vi "Get Switch Heater.vi"(2 "error in":T2, 3 "Communications Config":T1={"GPIB address"=22, "GPIB bus"=0, "connection ID"=refnum, "IP"="192.168.2.200", "Active Comm Interface"=0, "Serial Port"="", "Programmer Type"=0} {"Programmer Type" items=["Model 430", "Model 420"]; "Active Comm Interface" items=["TCP/IP (Model 430 Only)", "RS232", "IEEE488"]}) -> (0 "error out":T2, 1 "Switch Heater Indicator":bool)   [LabVIEW 2018]
panel:
  in  "GPIB Address":cluster{"GPIB address":i16, "GPIB bus":i16}={"GPIB address"=22, "GPIB bus"=0}
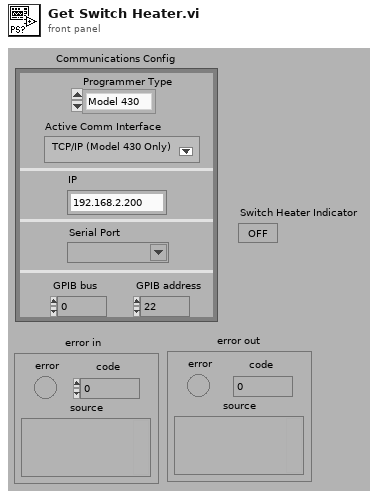
[diagram p1: front panel]
types:
  T1 = cluster{"GPIB address":i16, "GPIB bus":i16, "connection ID":refnum<k5>, "IP":string, "Active Comm Interface":u16, "Serial Port":refnum<visa-resource-name>, "Programmer Type":u16}
  T2 = cluster{"error":bool, "code":i32, "source":string}
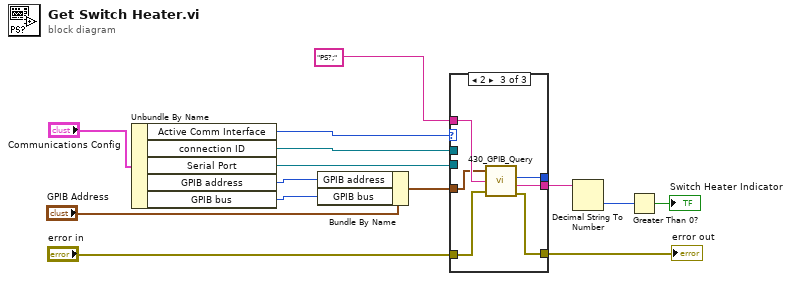
[diagram p0: block diagram]
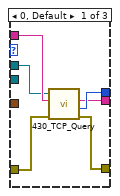
[diagram p2: hidden frame]
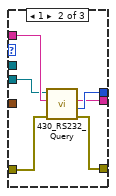
[diagram p3: hidden frame]
diagram:
  n1 = Unbundle By Name("Communications Config") -> ("Active Comm Interface"=w8:u16, "connection ID"=w7:refnum<k5>, "Serial Port"=w9:refnum<visa-resource-name>, "GPIB address"=w11:i16, "GPIB bus"=w12:i16)
  n2 = Bundle By Name(cluster="GPIB Address", "GPIB address"=w11, "GPIB bus"=w12) -> (w6:cluster{"GPIB address":i16, "GPIB bus":i16})
  n3 = case shown="2" w8 {
    tunnel: "PS?;" -> [w19 w25 w32]
    tunnel: "error in" -> [w15 w21 w31]
    tunnel: [w20 w26 w30] -> w4
    tunnel: [w17 w23 w28] -> w3
    tunnel: [w18 w24 w29] -> _
    tunnel: w9 -> [_ w22 _]
    tunnel: w7 -> [w16 _ _]
    tunnel: w6 -> [_ _ w27]
    frame 0, Default {
      n4 = call "430_TCP_Query.vi"("error in (no error)"=w15, "Command"=w19, "connection ID"=w16) -> ("error out"=w20:errorcluster, "Bytes Read"=w18:i32, "Response"=w17:string)  [unwired: 4 in, 2 out]
    }
    frame 1 {
      n5 = call "430_RS232_Query.vi"("error in (no error)"=w21, "Command"=w25, "VISA resource name"=w22) -> ("error out"=w26:errorcluster, "Bytes Read"=w24:i32, "Response"=w23:string)  [unwired: 4 in, 2 out]
    }
    frame 2 {
      n6 = call "430_GPIB_Query.vi"("GPIB (In)"=w27, "Input query"=w32, "error in"=w31) -> ("Bytes returned"=w29:i32, "Return string"=w28:string, "error out"=w30:T2)  [unwired: 1 out]
    }
  }
  "error out" <- w4
  n7 = Decimal String To Number(string=w3) -> (number=w14:i32)  [unwired: 2 in, 1 out]
  n8 = Greater Than 0?(x=w14) -> (x > 0?=→"Switch Heater Indicator":bool)
